vi "Get Destination Name.vi"(8 "error in (no error)":errorcluster, 10 "Default Destinations":T1(ring), 11 "SDIST in":refnum<class "NI_AB_API_DSDIST.lvclass">) -> (0 "error out":errorcluster, 2 "Destination Name":string, 3 "SDIST out":refnum<class "NI_AB_API_DSDIST.lvclass">)   [LabVIEW 2020, in "NI_AB_API_DSDIST.lvclass"]
uses:
  <vilib>/AppBuilder/AB_API/DSDIST/NI_AB_API_DSDIST.lvclass
  <vilib>/AppBuilder/AB_API/SDIST/NI_AB_API_SDIST.lvclass
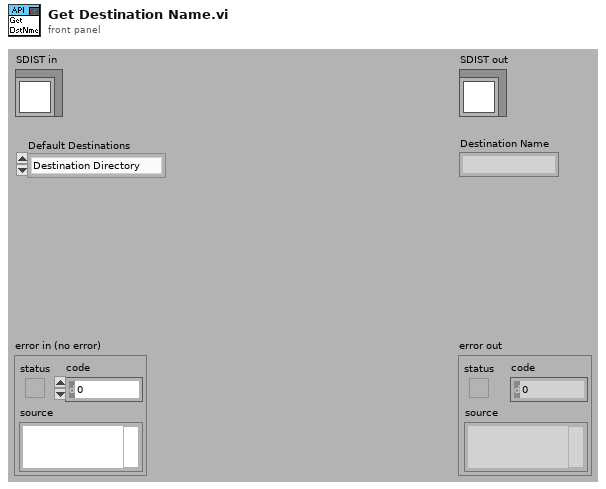
[diagram p1: front panel]
types:
  T1 = enum16{"Destination Directory", "Support Directory"}
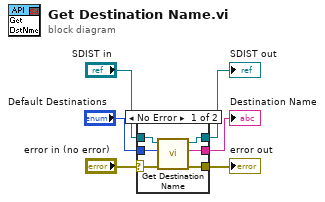
[diagram p0: block diagram]
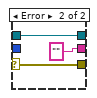
[diagram p2: hidden frame]
diagram:
  n1 = case shown="No Error" "error in (no error)" {
    selector: "error in (no error)" -> [w10 w15]
    tunnel: [w9 w15] -> w5
    tunnel: [w11 w14] -> w3
    tunnel: "SDIST in" -> [w12 w14]
    tunnel: "Default Destinations" -> [w7 _]
    tunnel: [w8 "" ("Destination Name")] -> w1
    frame No Error {
      n2 = call-parent "Get Destination Name.vi"("error in (no error)"=w10, "Default Destinations"=w7, "SDIST in"=w12) -> ("error out"=w9:errorcluster, "Destination Name"=w8:string, "SDIST out"=w11:refnum<class "NI_AB_API_DSDIST.lvclass">)  [unwired: 6 in]
    }
    frame Error {
    }
  }
  "error out" <- w5
  "SDIST out" <- w3
  "Destination Name" <- w1
